vi "Data Monitor.vi"(11 "Data":T1) -> (2 "Data Out":string, 3 "Identifier":string)   [LabVIEW 2020]
uses:
  Global/Data Global/SDQ Data Type.ctl
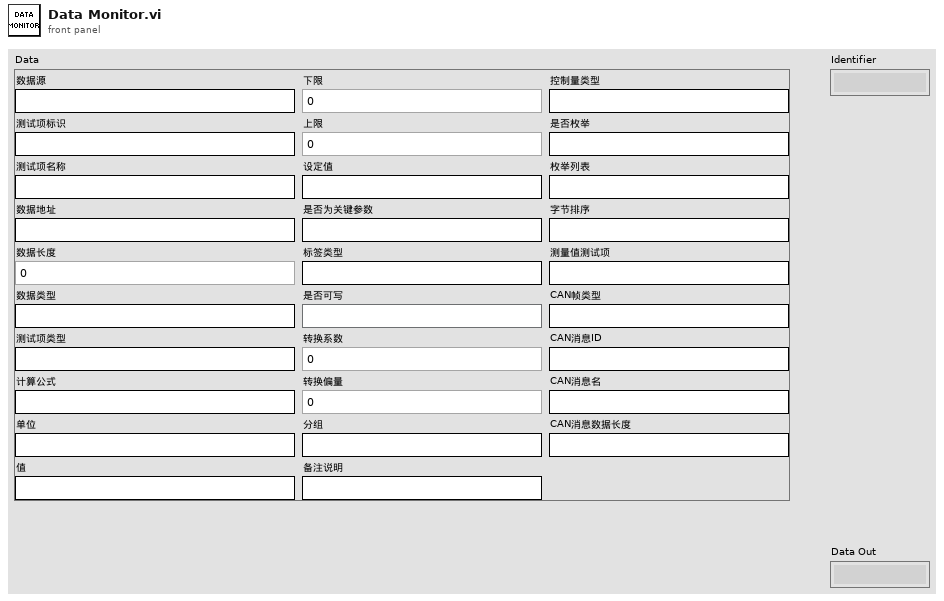
[diagram p1: front panel]
types:
  T1 = typedef "SDQ Data Type.ctl" = cluster{"CAN Length":string, "CAN Name":string, "CAN ID":string, "CAN Type":string, "Test Item":string, "Byte Order":string, "Instruction":string, "Control Type":string, "Group":string, "Offset":dbl, "Coefficient":dbl, "Write Enable":bool, "Lable Type":string, "Key?":string, "Set Value":string, "Upper":dbl, "Lower":dbl, "Unit":string, "Formula":string, "Test Item Type":string, "Length":i32, "Address":string, "Name":string, "Identifier":string, "Data Type":string, "Enumerate?":string, "Enumerate List":string, "Data":string, "Source":string}
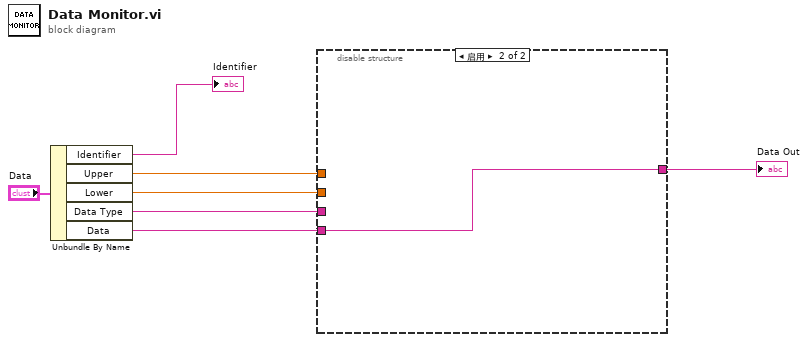
[diagram p0: block diagram]
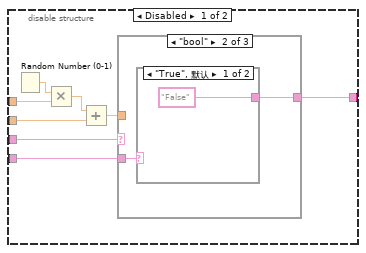
[diagram p2: hidden frame]
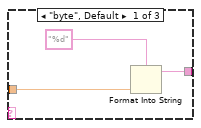
[diagram p3: hidden frame]
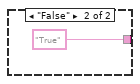
[diagram p4: hidden frame]
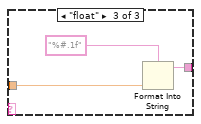
[diagram p5: hidden frame]
diagram:
  n1 = Unbundle By Name("Data") -> ("Identifier"=→"Identifier":string, "Upper"=w6:dbl, "Lower"=w7:dbl, "Data Type"=w3:string, "Data"=w2:string)
  n2 = disable-structure shown="启用" {
    disable-tunnel: w7 -> [w15 _]
    disable-tunnel: w6 -> [w13 _]
    disable-tunnel: w3 -> [w11 _]
    disable-tunnel: w2 -> [w10 w26]
    disable-tunnel: [w9 w26] -> w1
    frame Disabled {
      n3 = Random Number (0-1)() -> (number: 0 to 1=w14:dbl)
      n4 = Multiply(x=w14, y=w13) -> (x*y=w12:dbl)
      n5 = Add(x=w12, y=w15) -> (x+y=w8:dbl)
      n6 = case shown="\"bool\"" w11 {
        tunnel: w10 -> [_ w20 _]
        tunnel: [w16 w19 w23] -> w9
        tunnel: w8 -> [w17 _ w24]
        frame "byte", Default {
          n7 = Format Into String(format string="%d" ("格式字符串"), w17) -> (resulting string=w16:string)  [unwired: 2 in, 1 out]
        }
        frame "bool" {
          n8 = case shown="\"True\", 默认" w20 {
            tunnel: ["False" "True"] -> w19
            frame "True", Default {
            }
            frame "False" {
            }
          }
        }
        frame "float" {
          n9 = Format Into String(format string="%#.1f" ("格式字符串"), w24) -> (resulting string=w23:string)  [unwired: 2 in, 1 out]
        }
      }
    }
    frame Enabled {
    }
  }
  "Data Out" <- w1
